vi "Configure Burst Shape.vi"(0 "VISA resource name":refnum<visa-resource-name>, 1 "Rise Delay (0 bit)":dbl, 2 "Rise Time (10 bits)":dbl=10.0, 5 "Burst Shape (0: Sine)":u16(ring) items=["Sine", "Select File"], 7 "File Name (\"\")":string, 9 "Fall Time (10 bits)":dbl=10.0, 11 "error in (no error)":errorcluster, 12 "Fall Delay (0 bit)":dbl) -> (4 "VISA resource name out":refnum<visa-resource-name>, 15 "error out":errorcluster)   [LabVIEW 2014, in "Agilent PSG MXG Series.lvlib"]
doc: "Configures burst shape, rise time, rise delay, fall time and fall delay.\n\n<B>Notes:</B>\n(1) This VI is valid only in E8267C, E8267D, N5172B, N5182B.\n\n(2) For E8267C, this VI is valid only when the instrument installs <B>Option 002</B> (Internal baseband generator) or <B>Option 602</B> (Digital bus baseband generator).\n\n(3) For E8267D, this VI is valid only when the instrument installs <B>Option 601</B> or <B>Option 602</B> (Internal baseband generator).\n\n(4) For N5172B and N5182B, this VI is valid only when the instrument installs <B>Option 431</B>."
uses:
  Agilent PSG MXG Series.lvlib
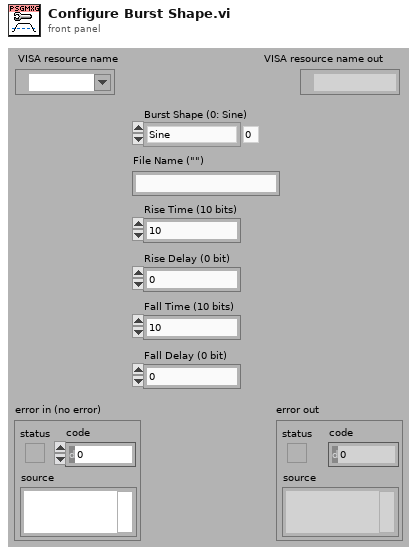
[diagram p1: front panel]
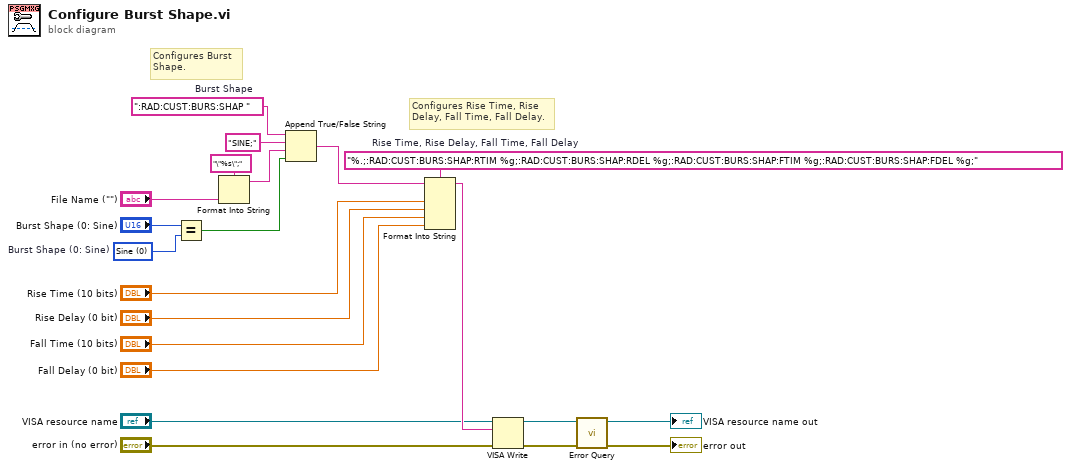
[diagram p0: block diagram]
diagram:
  w12 = "%.;:RAD:CUST:BURS:SHAP:RTIM %g;:RAD:CUST:BURS:SHAP:RDEL %g;:RAD:CUST:BURS:SHAP:FTIM %g;:RAD:CUST:BURS:SHAP:FDEL %g;"  # Rise Time, Rise Delay, Fall Time, Fall Delay
  w19 = ":RAD:CUST:BURS:SHAP "  # Burst Shape
  w20 = u16 0 items=["Sine", "Select File"]  # Burst Shape (0: Sine)
  # "Configures Rise Time, Rise\nDelay, Fall Time, Fall Delay."
  # "Configures Burst\nShape."
  n1 = Equal?(x="Burst Shape (0: Sine)", y=w20) -> (x = y?=w14:bool)
  n2 = Format Into String(format string="\"%s\";", "File Name (\"\")") -> (resulting string=w17:string)  [unwired: 2 in, 1 out]
  n3 = Append True/False String(1:w14, 2:w17, 3:"SINE;" ("true string"), 4:w19) -> (0:w13:string)
  n4 = Format Into String(format string=w12, initial string=w13, "Rise Time (10 bits)", "Rise Delay (0 bit)", "Fall Time (10 bits)", "Fall Delay (0 bit)") -> (resulting string=w7:string)  [unwired: 1 in, 1 out]
  n5 = VISA Write(VISA resource name="VISA resource name", write buffer=w7, error in (no error)="error in (no error)") -> (VISA resource name out=w6:refnum<visa-resource-name>, error out=w5:errorcluster)  [unwired: 1 out]
  n6 = call "Error Query.vi"("error in (no error)"=w5, "VISA resource name"=w6) -> ("error out"=→"error out":errorcluster, "VISA resource name out"=→"VISA resource name out":refnum<visa-resource-name>)  [unwired: 8 out]
